vi "Read Insertion Info.vi"(11 "Viewable in":refnum<class "IViewable.lvclass">) -> (1 "Name":string, 2 "VI Refnum":refnum<vi>, 3 "Viewable Callback Enqueuer":refnum<class "Message Enqueuer.lvclass">)   [LabVIEW 2020, in "IViewable.lvlib" / "IViewable.lvclass"]
doc: "读取插入信息"
uses:
  IViewable.lvclass
  C:/Program Files/National Instruments/LabVIEW 2020/vi.lib/ActorFramework/Actor/Actor.lvclass
  <vilib>/ActorFramework/Message Enqueuer/Message Enqueuer.lvclass
  <vilib>/ActorFramework/Actor/Actor.lvclass/Actor.ctl
  <vilib>/ActorFramework/Message Enqueuer/Message Enqueuer.lvclass/Message Enqueuer.ctl
  IViewable.lvclass/IViewable.ctl
  <vilib>/ActorFramework/Message Enqueuer/Init from Existing Queue.vi
  <vilib>/ActorFramework/Actor/Actor.lvclass
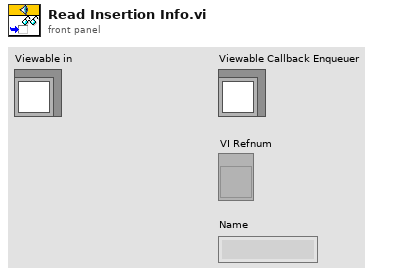
[diagram p1: front panel]
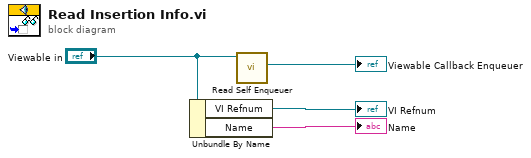
[diagram p0: block diagram]
diagram:
  n1 = Unbundle By Name("Viewable in") -> ("VI Refnum"=→"VI Refnum":refnum<vi>, "Name"=→"Name":string)
  n2 = call <vilib>:"Read Self Enqueuer.vi"("Actor"="Viewable in") -> ("Self Enqueuer"=→"Viewable Callback Enqueuer":refnum<class "Message Enqueuer.lvclass">)  [unwired: 10 in]
